vi "Expander Write.vi"(6 "NoStop (F)":bool, 8 "error in (no error)":errorcluster, 9 "Value":u8 format="%.0x", 10 "Session in":refnum<class "Session.lvclass">, 11 "PCF8574 I2C LCD in":refnum<class "PCF8574 I2C LCD.lvclass">) -> (0 "error out":errorcluster, 2 "Session out":refnum<class "Session.lvclass">, 3 "PCF8574 I2C LCD out":refnum<class "PCF8574 I2C LCD.lvclass">)   [LabVIEW 2020, in "CTI-Peripheral.lvlib" / "PCF8574 I2C LCD.lvclass"]
uses:
  PCF8574 I2C LCD.lvclass
  CTI/Session/Session.lvclass
  PCF8574 I2C LCD.lvclass/PCF8574 I2C LCD.ctl
  CTI/I2C Peripheral/I2C Peripheral.lvclass/I2C Peripheral.ctl
  CTI/Session/I2C Write Data.vi
  CTI/I2C Peripheral/I2C Peripheral.lvclass
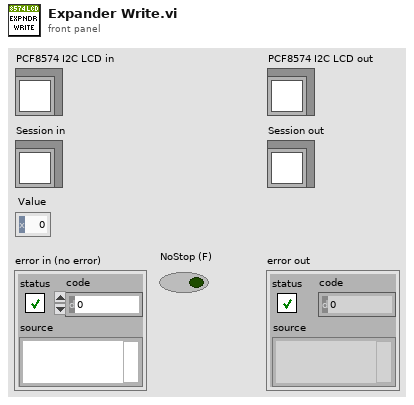
[diagram p1: front panel]
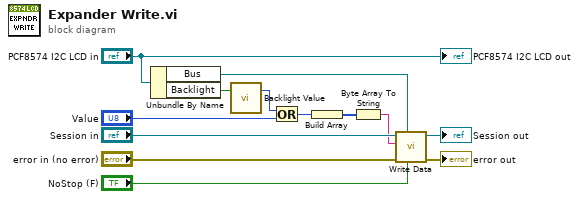
[diagram p0: block diagram]
diagram:
  n1 = Unbundle By Name("PCF8574 I2C LCD in") -> ("Bus"=w2:refnum<class "I2C Peripheral.lvclass">, "Backlight"=w11:bool)
  n2 = call "Backlight Value.vi"("Backlight"=w11) -> ("BacklightVal"=w10:u8)  [unwired: 2 in]
  n3 = Or(x=w10, y="Value") -> (x .or. y?=w9:u8)
  n4 = Build Array(w9) -> (w8:u8[])
  n5 = Byte Array To String(unsigned byte array=w8) -> (string=w3:string)
  n6 = call "Write Data.vi"("NoStop (F)"="NoStop (F)", "I2C Peripheral"=w2, "error in (no error)"="error in (no error)", "Data"=w3, "Session In"="Session in") -> ("error out"=→"error out":errorcluster, "Session Out"=→"Session out":refnum<class "Session.lvclass">)  [unwired: 5 in]
  "PCF8574 I2C LCD out" <- "PCF8574 I2C LCD in"
